vi "TestSeriellRT.vi"() -> ()   [LabVIEW 2010]
uses:
  <vilib>/LabVIEW Targets/FPGA/cRIO/shared/nicrio_ModuleControls/nicrio_cRIO-9871_BaudRateEnum.ctl
  <vilib>/LabVIEW Targets/FPGA/cRIO/shared/nicrio_ModuleControls/nicrio_cRIO-9871_DataBitsEnum.ctl
  <vilib>/LabVIEW Targets/FPGA/cRIO/shared/nicrio_ModuleControls/nicrio_cRIO-9871_ParityEnum.ctl
  <vilib>/LabVIEW Targets/FPGA/cRIO/shared/nicrio_ModuleControls/nicrio_cRIO-9871_StopBitsEnum.ctl
  <vilib>/LabVIEW Targets/FPGA/cRIO/shared/nicrio_ModuleControls/nicrio_cRIO-9871_FlowControlEnum.ctl
  <vilib>/userDefined/High Color/nirio_resource_hc.ctl
  <vilib>/rvi/interface/nirviOpenFPGA/nirviOpenFPGA.xnode
  C:/Users/HAGAR-IV/Desktop/Zeugs/markus/version feb 2012/FPGA Bitfiles/pertrasgcfpga2_FPGATarget_FPGA-Programm-11_875D3646.lvbitx
  C:/Users/HAGAR-IV/Desktop/Zeugs/Johnny/pertrasgc fpga/FPGA-Programm-11-15.vi
  <vilib>/rvi/ClientSDK/nirviWhatTheDeviceIsDoing.ctl
  <vilib>/rvi/interface/nirviReadWriteControl/nirviReadWriteControl.xnode
  <vilib>/rvi/interface/common/niFpgaNodeNameForErrorReporting.ctl
  <vilib>/rvi/errors/niLvFpgaWhatHappensToTopLevelVI.ctl
  <vilib>/rvi/interface/nirviMethod/nirviMethod.xnode
  <vilib>/rvi/interface/nirviCloseFPGA/nirviCloseFPGA.xnode
  <vilib>/FPGAPlugInAG/cRIO-9114/niLvFpga_Open_cRIO-9114.vi
  <vilib>/Utility/error.llb/Error Cluster From Error Code.vi
  <vilib>/rvi/errors/niLvFpgaAdjustHostInterfaceError.vi
  <vilib>/FPGAPlugInAG/cRIO-9114/niLvFpga_Close_cRIO-9114.vi
  NiFpgaLv.dll
panel:
  in  "senden?":bool
  in  "Anschluß":u8(ring)=1 items=["Mod7/Port1"=1, "Mod7/Port2"=2, "Mod7/Port3"=3, "Mod7/Port4"=4, "Mod8/Port1"=5, "Mod8/Port2"=6, "Mod8/Port3"=7, "Mod8/Port4"=8]
  in  "Write":string
  in  "Anschluß":i32(ring) items=["Mod7/Port1", "Mod7/Port2", "Mod7/Port3", "Mod7/Port4", "Mod8/Port1", "Mod8/Port2", "Mod8/Port3", "Mod8/Port4"]
  out "Read":string
  out "Read":string[](array[string])
  in  "Stopp":bool
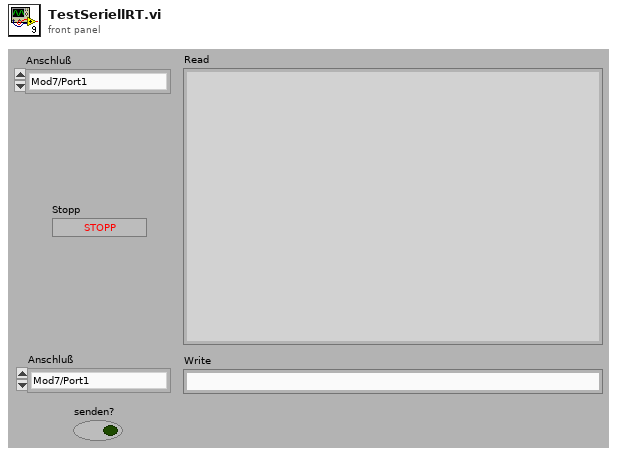
[diagram p1: front panel]
types:
  T1 = typedef "nicrio_cRIO-9871_BaudRateEnum.ctl" = enum16{"75 bps", "110 bps", "134 bps", "150 bps", "300 bps", "600 bps", "1200 bps", "1800 bps", "2400 bps", "4800 bps", "7200 bps", "9600 bps", "14.4 kbps", "19.2 kbps", "28.8 kbps", "38.4 kbps", "57.6 kbps", "115.2 kbps", "230.4 kbps", "460.8 kbps", "921.6 kbps"}
  T2 = typedef "nicrio_cRIO-9871_DataBitsEnum.ctl" = enum8{"5", "6", "7", "8"}
  T3 = typedef "nicrio_cRIO-9871_ParityEnum.ctl" = enum8{"None", "Odd", "Even", "Mark", "Space"}
  T4 = typedef "nicrio_cRIO-9871_StopBitsEnum.ctl" = enum8{"1", "1.5", "2"}
  T5 = typedef "nicrio_cRIO-9871_FlowControlEnum.ctl" = enum8{"None", "Software (XON / XOFF)", "Hardware (RTS / CTS)"}
  T6 = cluster{"Mod7/Port1":cluster{"Baud Rate":T1, "Data Bits":T2, "Parity":T3, "Stop Bits":T4, "Flow Control":T5}, "Mod7/Port2":cluster{"Baud Rate":T1, "Data Bits":T2, "Parity":T3, "Stop Bits":T4, "Flow Control":T5}, "Mod7/Port3":cluster{"Baud Rate":T1, "Data Bits":T2, "Parity":T3, "Stop Bits":T4, "Flow Control":T5}, "Mod7/Port4":cluster{"Baud Rate":T1, "Data Bits":T2, "Parity":T3, "Stop Bits":T4, "Flow Control":T5}, "Mod8/Port1":cluster{"Baud Rate":T1, "Data Bits":T2, "Parity":T3, "Stop Bits":T4, "Flow Control":T5}, "Mod8/Port2":cluster{"Baud Rate":T1, "Data Bits":T2, "Parity":T3, "Stop Bits":T4, "Flow Control":T5}, "Mod8/Port3":cluster{"Baud Rate":T1, "Data Bits":T2, "Parity":T3, "Stop Bits":T4, "Flow Control":T5}, "Mod8/Port4":cluster{"Baud Rate":T1, "Data Bits":T2, "Parity":T3, "Stop Bits":T4, "Flow Control":T5}}
  T7 = typedef "niFpgaNodeNameForErrorReporting.ctl" = enum16{"Open FPGA VI Reference", "Read/Write Control", "Invoke Method: Abort", "Invoke Method: Acknowledge IRQ", "Invoke Method: Download", "Invoke Method: FIFO.Configure", "Invoke Method: FIFO.Read", "Invoke Method: FIFO.Start", "Invoke Method: FIFO.Stop", "Invoke Method: FIFO.Write", "Invoke Method: Reset", "Invoke Method: Run", "Invoke Method: Wait on IRQ", "Close FPGA VI Reference"}
  T8 = typedef "niLvFpgaWhatHappensToTopLevelVI.ctl" = enum16{"top level VI scripted behind XNode", "top level VI inlined behind XNode"}
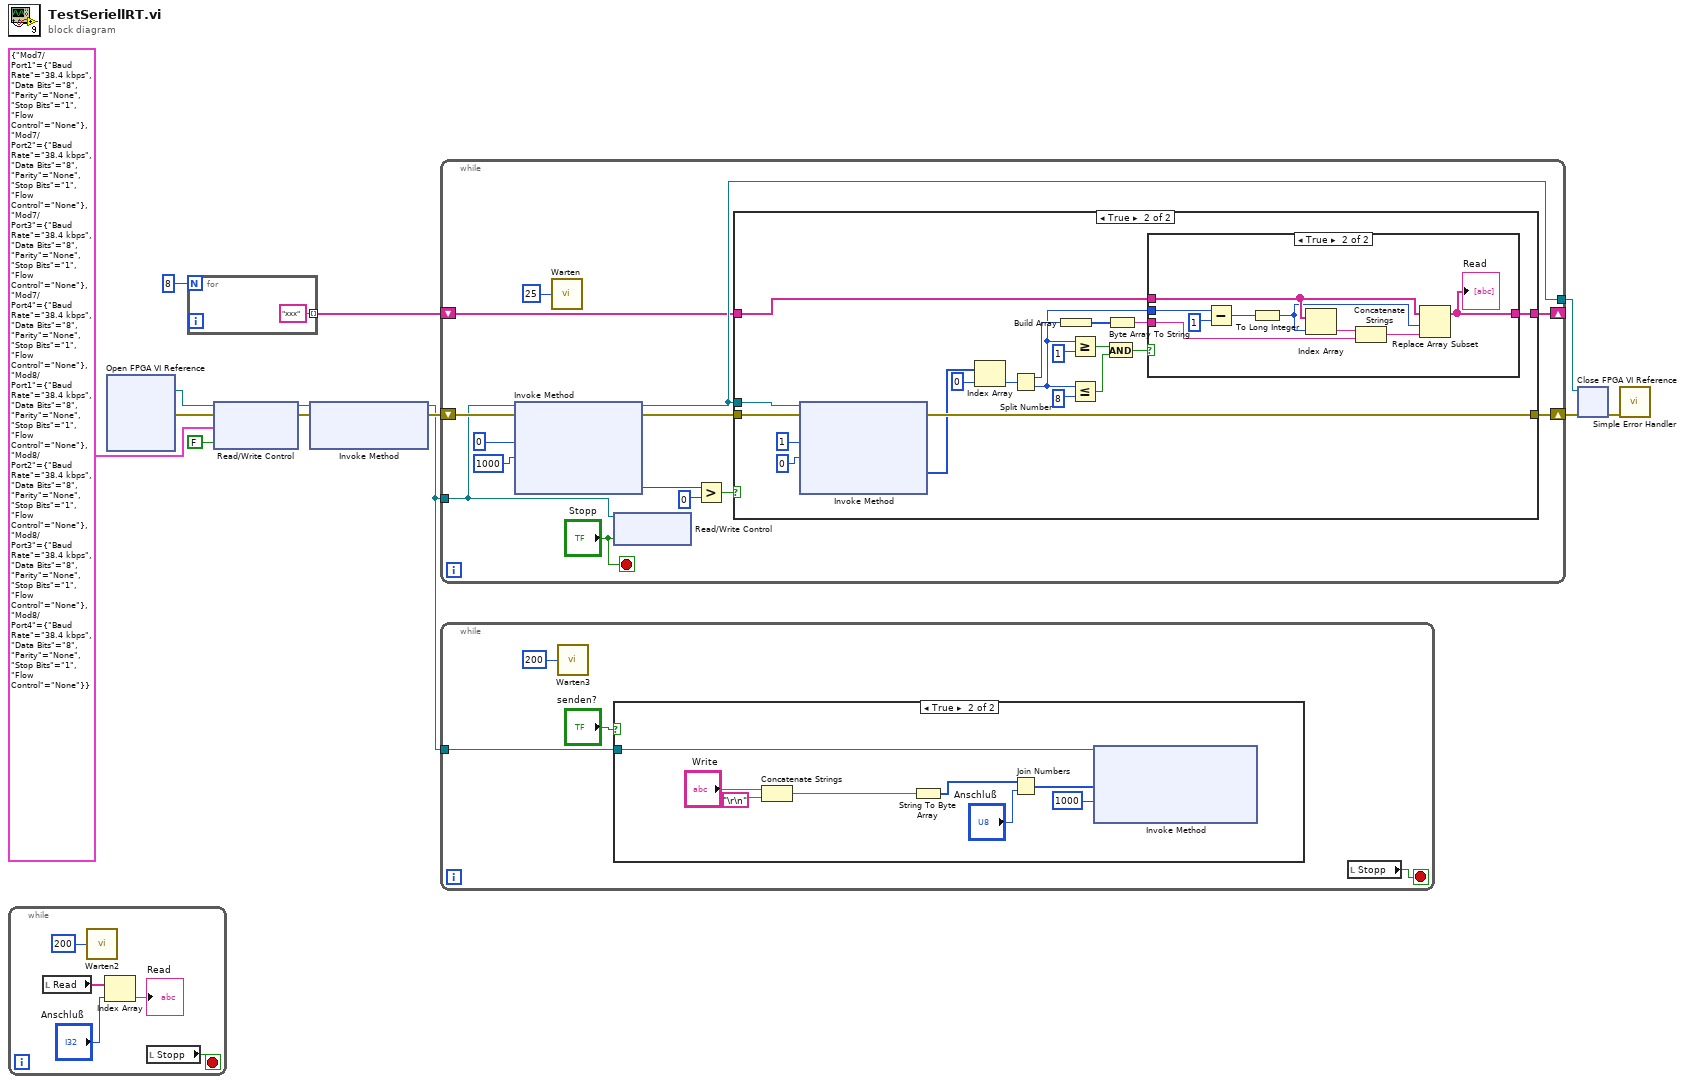
[diagram p0: block diagram]
diagram:
  n1 = while {
    stop <- w18 stop-if-true
    n2 = local read "Read"() -> (w17:string[])
    n3 = call "Warten2"("Count(mSec)"=u32 200) -> ()  [unwired: 1 out]
    n4 = Index Array(array=w17, index="Anschluß") -> (element=→"Read":string)
    n5 = local read "Stopp"() -> (w18:bool)
  }
  n6 = xnode "Open FPGA VI Reference"() -> ("FPGA VI Reference Out"=w13:refnum<k20>, "error out"=w12:errorcluster)  [unwired: 2 in]
  n7 = for {
    N: 8 -> [_]
    tunnel: ["xxx"] -> w2 mode=indexing
  }
  n8 = xnode "Read/Write Control"("FPGA VI Reference In"=w13, "error in"=w12, "KonfigSeriell"=T6 {"Mod7/Port1"={"Baud Rate"=enum."38.4 kbps", "Data Bits"=enum."8", "Parity"=enum."None", "Stop Bits"=enum."1", "Flow Control"=enum."None"}, "Mod7/Port2"={"Baud Rate"=enum."38.4 kbps", "Data Bits"=enum."8", "Parity"=enum."None", "Stop Bits"=enum."1", "Flow Control"=enum."None"}, "Mod7/Port3"={"Baud Rate"=enum."38.4 kbps", "Data Bits"=enum."8", "Parity"=enum."None", "Stop Bits"=enum."1", "Flow Control"=enum."None"}, "Mod7/Port4"={"Baud Rate"=enum."38.4 kbps", "Data Bits"=enum."8", "Parity"=enum."None", "Stop Bits"=enum."1", "Flow Control"=enum."None"}, "Mod8/Port1"={"Baud Rate"=enum."38.4 kbps", "Data Bits"=enum."8", "Parity"=enum."None", "Stop Bits"=enum."1", "Flow Control"=enum."None"}, "Mod8/Port2"={"Baud Rate"=enum."38.4 kbps", "Data Bits"=enum."8", "Parity"=enum."None", "Stop Bits"=enum."1", "Flow Control"=enum."None"}, "Mod8/Port3"={"Baud Rate"=enum."38.4 kbps", "Data Bits"=enum."8", "Parity"=enum."None", "Stop Bits"=enum."1", "Flow Control"=enum."None"}, "Mod8/Port4"={"Baud Rate"=enum."38.4 kbps", "Data Bits"=enum."8", "Parity"=enum."None", "Stop Bits"=enum."1", "Flow Control"=enum."None"}}, "global stop"=FALSE ("Stopp")) -> ("FPGA VI Reference Out"=w11:refnum<k20>, "error out"=w10:errorcluster)
  n9 = xnode "Invoke Method"("FPGA VI Reference In"=w11, "error in"=w10) -> ("FPGA VI Reference Out"=w1:refnum<k20>, "error out"=w6:errorcluster)  [unwired: 1 in]
  n10 = while {
    tunnel: w1 -> [w29]
    shift-right: [w22] -> w4
    shift-left: w6 -> [w31]
    shift-right: [w20] -> _
    shift-left: w2 -> [w21]
    tunnel: [w24] -> w5
    stop <- "Stopp" stop-if-true
    n11 = xnode "Invoke Method"("FPGA VI Reference In"=w29, "error in"=w31, "Number of Elements"=u32 0, "Timeout (ms)"=1000) -> ("FPGA VI Reference Out"=w24:refnum<k20>, "error out"=w23:errorcluster, "Elements Remaining"=w27:u32)  [unwired: 1 out]
    n12 = call "Warten"("Count(uSec)"=u32 25) -> ()  [unwired: 1 out]
    n13 = xnode "Read/Write Control"("FPGA VI Reference In"=w29, "global stop"="Stopp") -> ()  [unwired: 1 in, 2 out]
    n14 = Greater?(x=w27, y=u32 0) -> (0:w25:bool)
    n15 = case shown="True" w25 {
      tunnel: w21 -> [w34 w49]
      tunnel: [w34 w48] -> w20
      tunnel: w24 -> [_ w47]
      tunnel: w23 -> [w35 w46]
      tunnel: [w35 w45] -> w22
      frame False {
      }
      frame True {
        n16 = xnode "Invoke Method"("FPGA VI Reference In"=w47, "error in"=w46, "Number of Elements"=u32 1, "Timeout (ms)"=0) -> ("error out"=w45:errorcluster, "Data"=w43:u16[])  [unwired: 2 out]
        n17 = Index Array(array=w43, index=0 ("Index")) -> (element=w53:u16)
        n18 = Split Number(x=w53) -> (hi(x)=w52:u8, lo(x)=w40:u8)
        n19 = Build Array(w52) -> (w51:u8[])
        n20 = Greater Or Equal?(x=w40, y=u8 1) -> (x >= y?=w38:bool)
        n21 = Less Or Equal?(x=w40, y=u8 8) -> (x <= y?=w37:bool)
        n22 = And(x=w38, y=w37) -> (x .and. y?=w36:bool)
        n23 = Byte Array To String(unsigned byte array=w51) -> (string=w50:string)
        n24 = case shown="True" w36 {
          tunnel: w50 -> [_ w136]
          tunnel: w49 -> [w127 w131]
          tunnel: [w127 w128] -> w48
          tunnel: w40 -> [_ w135]
          frame False {
          }
          frame True {
            n25 = Subtract(x=w135, y=u8 1) -> (x-y=w133:u8)
            n26 = To Long Integer(number=w133) -> (32bit integer=w130:i32)
            n27 = Index Array(array=w131, index=w130) -> (element=w132:string)
            n28 = Concatenate Strings(w132, w136) -> (w129:string)
            n29 = Replace Array Subset(array=w131, new element=w129, index=w130) -> (w128:string[])
            "Read" <- w128
          }
        }
      }
    }
  }
  n30 = while {
    tunnel: w1 -> [w249]
    stop <- w250 stop-if-true
    n31 = call "Warten3"("Count(mSec)"=u32 200) -> ()  [unwired: 1 out]
    n32 = case shown="True" "senden?" {
      tunnel: w249 -> [_ w258]
      frame False {
      }
      frame True {
        n33 = Concatenate Strings("Write", "\r\n") -> (w251:string)
        n34 = String To Byte Array(string=w251) -> (unsigned byte array=w257:u8[])
        n35 = Join Numbers(hi=w257, lo="Anschluß") -> ((hi.lo)=w255:u16[])
        n36 = xnode "Invoke Method"("FPGA VI Reference In"=w258, "Data"=w255, "Timeout (ms)"=1000) -> ()  [unwired: 1 in, 3 out]
      }
    }
    n37 = local read "Stopp"() -> (w250:bool)
  }
  n38 = xnode "Close FPGA VI Reference"("FPGA VI Reference In"=w5, "error in"=w4) -> ("error out"=w9:errorcluster)
  n39 = call <vilib>:"Simple Error Handler.vi"("error in (no error)"=w9) -> ()  [unwired: 4 in, 5 out]
